vi "ReadFromSelectedChannel.vi"(0 "reference out 3":refnum<visa-resource-name>, 1 "error out":errorcluster) -> (2 "reference out 4":refnum<visa-resource-name>, 3 "read buffer":string, 4 "error out 2":errorcluster)   [LabVIEW 2009]
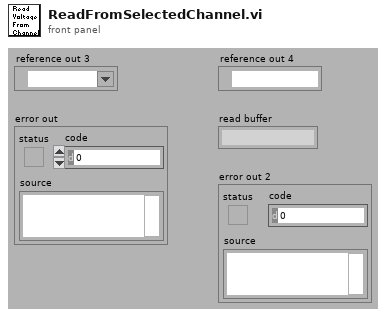
[diagram p1: front panel]
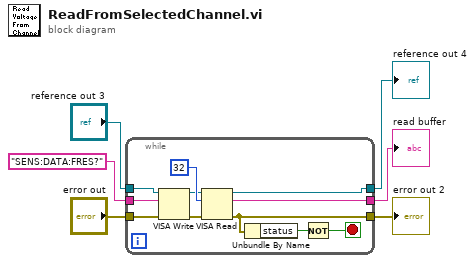
[diagram p0: block diagram]
diagram:
  n1 = while {
    tunnel: "error out" -> [w17]
    tunnel: "reference out 3" -> [w16]
    tunnel: [w15] -> w4
    tunnel: [w9] -> w3
    tunnel: [w14] -> w2
    tunnel: "SENS:DATA:FRES?" ("write buffer") -> [w10]
    stop <- w7 stop-if-true
    n2 = VISA Write(VISA resource name=w16, write buffer=w10, error in (no error)=w17) -> (VISA resource name out=w12:refnum<visa-resource-name>, error out=w11:errorcluster)  [unwired: 1 out]
    n3 = VISA Read(VISA resource name=w12, byte count=u32 32, error in (no error)=w11) -> (VISA resource name out=w14:refnum<visa-resource-name>, read buffer=w15:string, error out=w9:errorcluster)  [unwired: 1 out]
    n4 = Unbundle By Name(w9) -> ("status"=w8:bool)
    n5 = Not(x=w8) -> (.not. x?=w7:bool)
  }
  "read buffer" <- w4
  "error out 2" <- w3
  "reference out 4" <- w2
